vi "Format Variant.vi"(10 "Value":variant, 11 "Log Message":string) -> (0 "Error Out":errorcluster, 3 "Message":string)   [LabVIEW 2017, in "Composed Log.lvlib" / "LoggerReference.lvclass"]
uses:
  LoggerReference.lvclass
  <vilib>/Utility/Data Type/NI_Data Type.lvlib
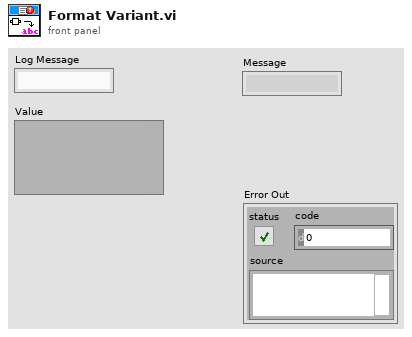
[diagram p1: front panel]
types:
  T1 = typedef "NI_Data Type.lvlib/Data Type.ctl" = enum8{"Invalid Type", "Void", "I8", "I16", "I32", "I64", "U8", "U16", "U32", "U64", "Single Float", "Double Float", "Extended Float", "Single Complex", "Double Complex", "Extended Complex", "Enum U8", "Enum U16", "Enum U32", "Enum U64", "Single Float With Unit", "Double Float With Unit", "Extended Float With Unit", "Single Complex with Unit", "Double Complex with Unit", "Extended Complex with Unit", "Boolean", "String", "Path", "Picture", "Tag", "Array", "Cluster", "Variant", "LV Variant", "Waveform", "Timestamp", "Digital Waveform", "Digital Data", "ExpressData", "Refnum", "External Data", "VI", "Poly VI", "LabVIEW Class Instance", "Fixed Point"}
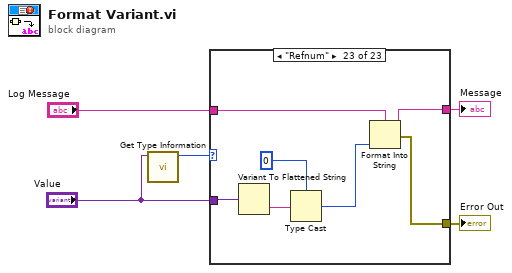
[diagram p0: block diagram]
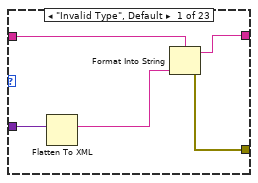
[diagram p2: hidden frame]
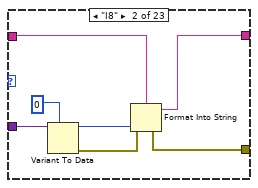
[diagram p3: hidden frame]
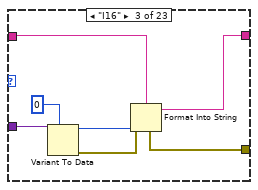
[diagram p4: hidden frame]
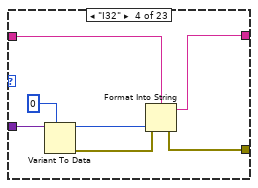
[diagram p5: hidden frame]
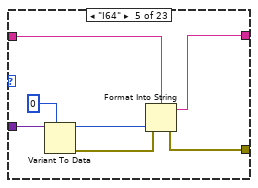
[diagram p6: hidden frame]
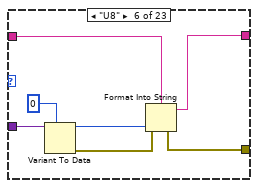
[diagram p7: hidden frame]
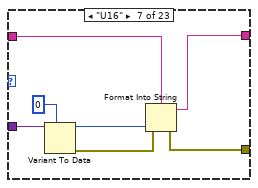
[diagram p8: hidden frame]
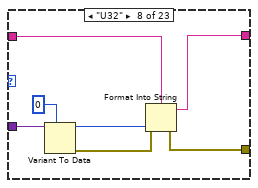
[diagram p9: hidden frame]
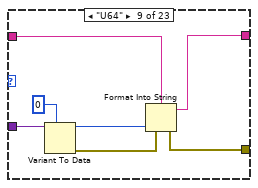
[diagram p10: hidden frame]
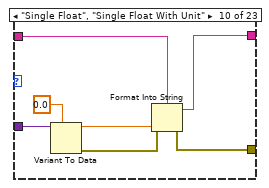
[diagram p11: hidden frame]
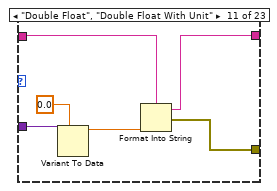
[diagram p12: hidden frame]
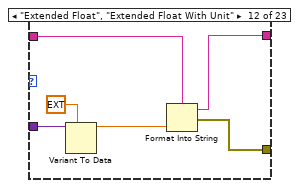
[diagram p13: hidden frame]
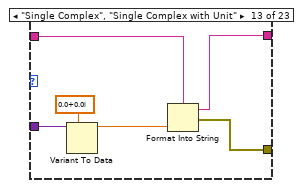
[diagram p14: hidden frame]
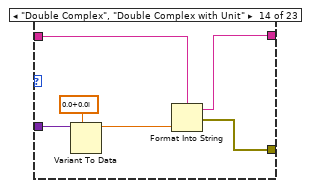
[diagram p15: hidden frame]
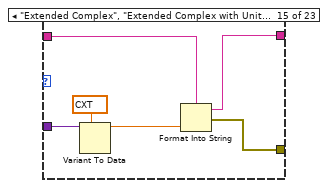
[diagram p16: hidden frame]
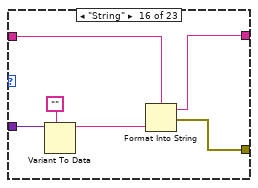
[diagram p17: hidden frame]
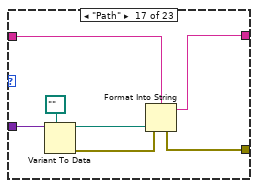
[diagram p18: hidden frame]
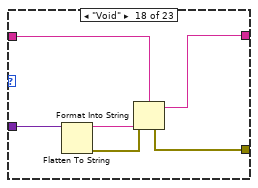
[diagram p19: hidden frame]
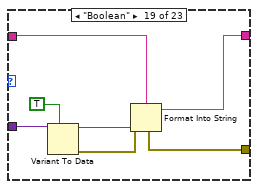
[diagram p20: hidden frame]
diagram:
  n1 = call <vilib>:"Get Type Information.vi"("Variant"="Value") -> ("Type"=w5:T1)  [unwired: 6 in, 4 out]
  n2 = case shown="\"Refnum\"" w5 {
    tunnel: "Log Message" -> [w6 w14 w21 w29 w36 w43 w50 w57 w64 w71 w76 w83 w89 w95 w101 w107 w114 w122 w126 w137 w142 w150 w156]
    tunnel: [w9 w13 w20 w27 w34 w41 w48 w55 w62 w69 w75 w81 w87 w93 w99 w105 w112 w121 w125 w136 w140 w149 w155] -> w2
    tunnel: "Value" -> [w10 w17 w24 w31 w38 w45 w52 w59 w66 w73 w79 w85 w91 w97 w103 w109 w116 w119 w129 w135 w146 w153 w160]
    tunnel: [w7 w12 w19 w26 w33 w40 w47 w54 w61 w68 w74 w80 w86 w92 w98 w104 w111 w118 w124 w130 w138 w147 w154] -> w1
    frame "Invalid Type", Default {
      n3 = Flatten To XML(anything=w10) -> (xml string=w8:string)
      n4 = Format Into String(format string=w6, w8) -> (resulting string=w9:string, error out=w7:errorcluster)  [unwired: 2 in]
    }
    frame "I8" {
      n5 = Variant To Data(type=i8 0, Variant=w17) -> (data=w15:i8, error out=w11:errorcluster)  [unwired: 1 in]
      n6 = Format Into String(format string=w14, error in=w11, w15) -> (resulting string=w13:string, error out=w12:errorcluster)  [unwired: 1 in]
    }
    frame "I16" {
      n7 = Variant To Data(type=i16 0, Variant=w24) -> (data=w22:i16, error out=w18:errorcluster)  [unwired: 1 in]
      n8 = Format Into String(format string=w21, error in=w18, w22) -> (resulting string=w20:string, error out=w19:errorcluster)  [unwired: 1 in]
    }
    frame "I32" {
      n9 = Variant To Data(type=0, Variant=w31) -> (data=w28:i32, error out=w25:errorcluster)  [unwired: 1 in]
      n10 = Format Into String(format string=w29, error in=w25, w28) -> (resulting string=w27:string, error out=w26:errorcluster)  [unwired: 1 in]
    }
    frame "I64" {
      n11 = Variant To Data(type=i64 0, Variant=w38) -> (data=w35:i64, error out=w32:errorcluster)  [unwired: 1 in]
      n12 = Format Into String(format string=w36, error in=w32, w35) -> (resulting string=w34:string, error out=w33:errorcluster)  [unwired: 1 in]
    }
    frame "U8" {
      n13 = Variant To Data(type=u8 0, Variant=w45) -> (data=w42:u8, error out=w39:errorcluster)  [unwired: 1 in]
      n14 = Format Into String(format string=w43, error in=w39, w42) -> (resulting string=w41:string, error out=w40:errorcluster)  [unwired: 1 in]
    }
    frame "U16" {
      n15 = Variant To Data(type=u16 0, Variant=w52) -> (data=w49:u16, error out=w46:errorcluster)  [unwired: 1 in]
      n16 = Format Into String(format string=w50, error in=w46, w49) -> (resulting string=w48:string, error out=w47:errorcluster)  [unwired: 1 in]
    }
    frame "U32" {
      n17 = Variant To Data(type=u32 0, Variant=w59) -> (data=w56:u32, error out=w53:errorcluster)  [unwired: 1 in]
      n18 = Format Into String(format string=w57, error in=w53, w56) -> (resulting string=w55:string, error out=w54:errorcluster)  [unwired: 1 in]
    }
    frame "U64" {
      n19 = Variant To Data(type=u64 0, Variant=w66) -> (data=w63:u64, error out=w60:errorcluster)  [unwired: 1 in]
      n20 = Format Into String(format string=w64, error in=w60, w63) -> (resulting string=w62:string, error out=w61:errorcluster)  [unwired: 1 in]
    }
    frame "Single Float", "Single Float With Unit" {
      n21 = Variant To Data(type=sgl 0.0, Variant=w73) -> (data=w70:sgl, error out=w67:errorcluster)  [unwired: 1 in]
      n22 = Format Into String(format string=w71, error in=w67, w70) -> (resulting string=w69:string, error out=w68:errorcluster)  [unwired: 1 in]
    }
    frame "Double Float", "Double Float With Unit" {
      n23 = Variant To Data(type=0.0, Variant=w79) -> (data=w77:dbl)  [unwired: 1 in, 1 out]
      n24 = Format Into String(format string=w76, w77) -> (resulting string=w75:string, error out=w74:errorcluster)  [unwired: 2 in]
    }
    frame "Extended Float", "Extended Float With Unit" {
      n25 = Variant To Data(type=ext 0.0, Variant=w85) -> (data=w82:ext)  [unwired: 1 in, 1 out]
      n26 = Format Into String(format string=w83, w82) -> (resulting string=w81:string, error out=w80:errorcluster)  [unwired: 2 in]
    }
    frame "Single Complex", "Single Complex with Unit" {
      n27 = Variant To Data(type=csg 0.0+0.0i, Variant=w91) -> (data=w88:csg)  [unwired: 1 in, 1 out]
      n28 = Format Into String(format string=w89, w88) -> (resulting string=w87:string, error out=w86:errorcluster)  [unwired: 2 in]
    }
    frame "Double Complex", "Double Complex with Unit" {
      n29 = Variant To Data(type=cdb 0.0+0.0i, Variant=w97) -> (data=w94:cdb)  [unwired: 1 in, 1 out]
      n30 = Format Into String(format string=w95, w94) -> (resulting string=w93:string, error out=w92:errorcluster)  [unwired: 2 in]
    }
    frame "Extended Complex", "Extended Complex with Unit" {
      n31 = Variant To Data(type=cxt 0.0+0.0i, Variant=w103) -> (data=w100:cxt)  [unwired: 1 in, 1 out]
      n32 = Format Into String(format string=w101, w100) -> (resulting string=w99:string, error out=w98:errorcluster)  [unwired: 2 in]
    }
    frame "String" {
      n33 = Variant To Data(type="", Variant=w109) -> (data=w106:string)  [unwired: 1 in, 1 out]
      n34 = Format Into String(format string=w107, w106) -> (resulting string=w105:string, error out=w104:errorcluster)  [unwired: 2 in]
    }
    frame "Path" {
      n35 = Variant To Data(type=path "", Variant=w116) -> (data=w113:path, error out=w110:errorcluster)  [unwired: 1 in]
      n36 = Format Into String(format string=w114, error in=w110, w113) -> (resulting string=w112:string, error out=w111:errorcluster)  [unwired: 1 in]
    }
    frame "Void" {
      n37 = Flatten To String(anything=w119) -> (data string=w120:string, error out=w117:errorcluster)  [unwired: 3 in, 1 out]
      n38 = Format Into String(format string=w122, error in=w117, w120) -> (resulting string=w121:string, error out=w118:errorcluster)  [unwired: 1 in]
    }
    frame "Boolean" {
      n39 = Variant To Data(type=TRUE, Variant=w129) -> (data=w127:bool, error out=w123:errorcluster)  [unwired: 1 in]
      n40 = Format Into String(format string=w126, error in=w123, w127) -> (resulting string=w125:string, error out=w124:errorcluster)  [unwired: 1 in]
    }
    frame "LabVIEW Class Instance" {
      n41 = Variant To Data(type=refnum<class> refnum ("LabVIEW Object"), Variant=w135) -> (data=w133:refnum<class>, error out=w131:errorcluster)  [unwired: 1 in]
      n42 = Flatten To XML(anything=w133) -> (xml string=w132:string)
      n43 = Format Into String(format string=w137, error in=w131, w132) -> (resulting string=w136:string, error out=w130:errorcluster)  [unwired: 1 in]
    }
    frame "Enum U8".."Enum U64" {
      n44 = Variant To Data(type=u64 0, Variant=w146) -> (data=w143:u64, error out=w139:errorcluster)  [unwired: 1 in]
      n45 = call <vilib>:"Get Numeric Information.vi"("Variant"=w146) -> ("Enum Names"=w144:string[])  [unwired: 7 in, 3 out]
      n46 = Index Array(array=w144, index=w143) -> (element=w141:string)
      n47 = Format Into String(format string=w142, error in=w139, w141) -> (resulting string=w140:string, error out=w138:errorcluster)  [unwired: 1 in]
    }
    frame "Timestamp" {
      n48 = Variant To Data(type=timestamp(0 s since 1904-01-01), Variant=w153) -> (data=w151:timestamp, error out=w148:errorcluster)  [unwired: 1 in]
      n49 = Format Into String(format string=w150, error in=w148, w151) -> (resulting string=w149:string, error out=w147:errorcluster)  [unwired: 1 in]
    }
    frame "Refnum" {
      n50 = Variant To Flattened String(Variant=w160) -> (data string=w159:string)  [unwired: 1 out]
      n51 = Type Cast(type=0, x=w159) -> (*(type *) &x=w157:i32)
      n52 = Format Into String(format string=w156, w157) -> (resulting string=w155:string, error out=w154:errorcluster)  [unwired: 2 in]
    }
  }
  "Message" <- w2
  "Error Out" <- w1
